vi "Set Write Access.vi"(8 "error in (no error)":errorcluster, 10 "Write Access":enum8{"Allowed", "Required", "None"}(ring), 11 "abs_SharedVar_Bool in":refnum<class "conc_SharedVar_Bool.lvclass">) -> (0 "error out":errorcluster, 3 "abs_SharedVar_Bool out":refnum<class "conc_SharedVar_Bool.lvclass">)   [LabVIEW 2021, in "conc_SharedVar_Bool.lvclass"]
doc: "LVabs_Shared Variable 1.0.0.2\nTim - TSA\nCopyright (c) 2024, TSA"
uses:
  conc_SharedVar_Bool.lvclass
  conc_SharedVar_Bool.lvclass/conc_SharedVar_Bool.ctl
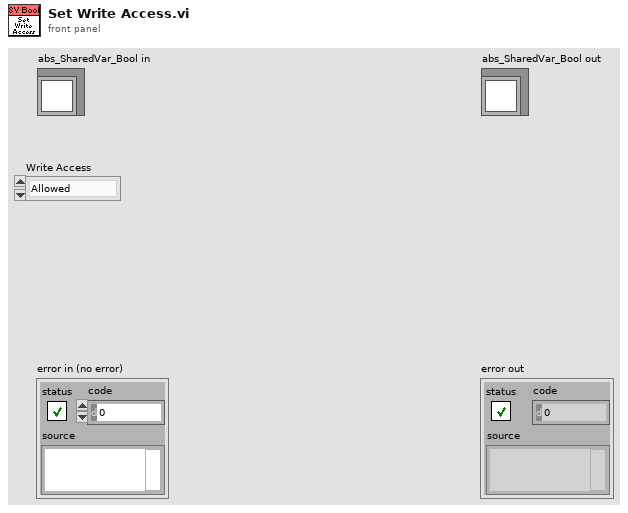
[diagram p1: front panel]
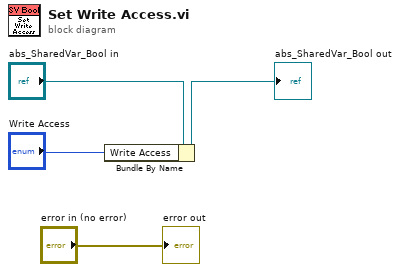
[diagram p0: block diagram]
diagram:
  n1 = Bundle By Name(cluster="abs_SharedVar_Bool in", "Write Access"="Write Access") -> (→"abs_SharedVar_Bool out":refnum<class "conc_SharedVar_Bool.lvclass">)
  "error out" <- "error in (no error)"
